vi "Re-Anchor steps TreeItem.vi"(10 "indent (i=0)":i32, 11 "TreeItems":T1[](array[typedef])) -> (3 "TreeItems":T1[](array[typedef]))   [LabVIEW 2020, in "BetterDragAndDrop.lvlib" / "BetterTreeHandle.lvclass"]
uses:
  BetterTreeHandle/BetterTreeHandle.lvclass
  TreeItem.ctl
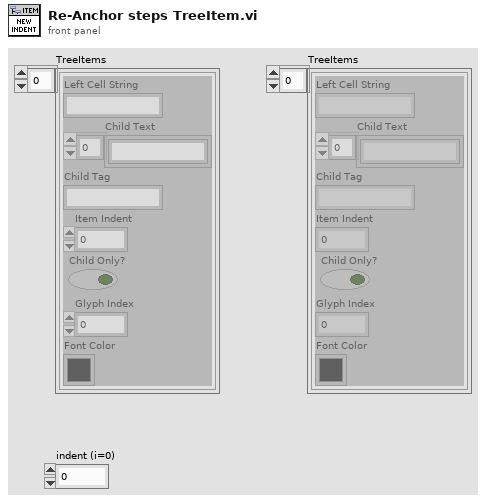
[diagram p1: front panel]
types:
  T1 = typedef "BetterDragAndDrop.lvlib/BetterTreeHandle.lvclass/TreeItem.ctl" = cluster{"Left Cell String":string, "Child Text":string[], "Child Tag":string, "Item Indent":i32, "Child Only?":bool, "Glyph Index":i32, "Font Color":u32}
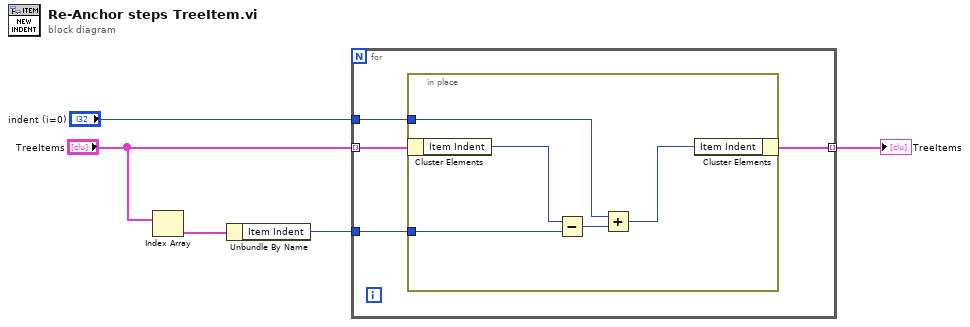
[diagram p0: block diagram]
diagram:
  n1 = Index Array(array="TreeItems") -> (element=w3:T1)  [unwired: 1 in]
  n2 = Unbundle By Name(w3) -> ("Item Indent"=w2:i32)
  n3 = for {
    tunnel: "TreeItems" -> [w7] mode=indexing
    tunnel: w2 -> [w9]
    tunnel: "indent (i=0)" -> [w8]
    tunnel: [w6] -> w1 mode=indexing
    n4 = in-place {
      in-place-border: w9 -> [w14]
      in-place-border: w8 -> [w12]
      n5 = in-place-cluster #1(w7) -> ("Item Indent"=w11:i32)
      n6 = Subtract(x=w11, y=w14) -> (x-y=w13:i32)
      n7 = Add(x=w12, y=w13) -> (x+y=w10:i32)
      n8 = in-place-cluster #1("Item Indent"=w10) -> (w6:T1)
    }
  }
  "TreeItems" <- w1
